vi "Method.vi"(4 "Input B":refnum<class "Abs_Numeric.lvclass">, 5 "Input A":refnum<class "Abs_Time.lvclass">) -> (1 "Result":refnum<class "Abs_Time.lvclass">)   [LabVIEW 2021, in "Subtract_Time.lvclass"]
uses:
  Subtract_Time.lvclass
  Abs_Types/Numeric/Abs_Numeric.lvclass
  Abs_Types/Time/Abs_Time.lvclass
  C:/Program Files (x86)/National Instruments/LabVIEW 2021/vi.lib/TSA/Abstract Data Classes/Abs_Types/Time/Abs_Time.lvclass
  Subtract_Time.lvclass/Subtract_Time.ctl
  Properties/Write Input A.vi
  Properties/Write Input B.vi
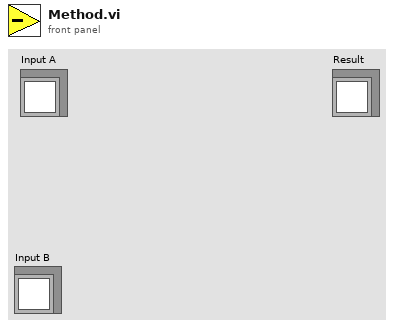
[diagram p1: front panel]
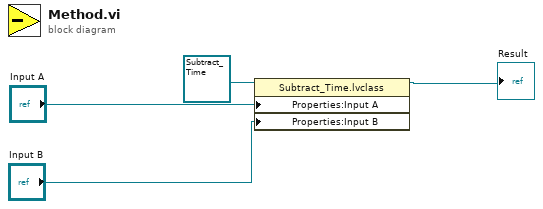
[diagram p0: block diagram]
diagram:
  n1 = property class="Subtract_Time.lvclass"(reference=refnum<class "Subtract_Time.lvclass"> refnum ("Subtract_DBL.lvclass"), "Properties:Input A"="Input A", "Properties:Input B"="Input B") -> (reference out=→"Result":refnum<class "Subtract_Time.lvclass">)  [unwired: 1 in, 1 out]
